vi "MB register buffer.vi"(8 "command":T1, 10 "Register number":dbl, 11 "register array in":cluster{"last read (s)":dbl, "last value":dbl[]}) -> (2 "last read (s)":dbl, 3 "register value":dbl)   [LabVIEW 2019]
uses:
  MB buffer cmd.ctl
panel:
  out "register array display":cluster{"last read (s)":dbl, "last value":dbl[]}
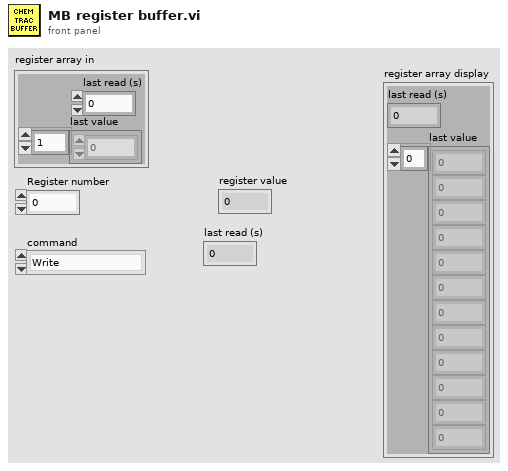
[diagram p1: front panel]
types:
  T1 = typedef "MB buffer cmd.ctl" = enum16{"Write", "Read", "Reset"}
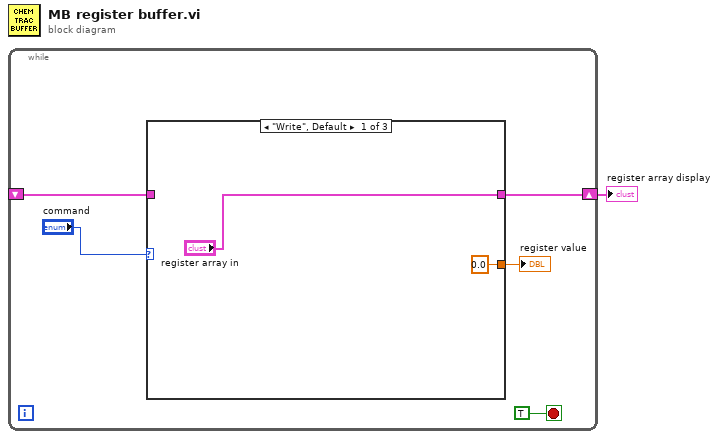
[diagram p0: block diagram]
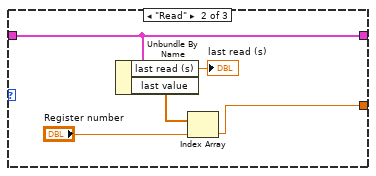
[diagram p2: hidden frame]
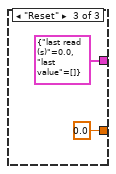
[diagram p3: hidden frame]
diagram:
  n1 = while {
    shift-right: [w4] -> w1
    shift-left: _ -> [w3]
    stop <- TRUE stop-if-true
    n2 = case shown="\"Write\", Default" "command" {
      tunnel: ["register array in" w13 cluster{"last read (s)":dbl, "last value":dbl[]} {"last read (s)"=0.0, "last value"=[]} ("register array in")] -> w4
      tunnel: w3 -> [_ w13 _]
      tunnel: [0.0 ("last value") w10 0.0 ("last value")] -> w2
      frame "Write", Default {
      }
      frame "Read" {
        n3 = Unbundle By Name(w13) -> ("last read (s)"=→"last read (s)":dbl, "last value"=w12:dbl[])
        n4 = Index Array(array=w12, index="Register number") -> (element=w10:dbl)
      }
      frame "Reset" {
      }
    }
    "register value" <- w2
  }
  "register array display" <- w1
